vi "Test 2 Degenerate Case Arrangement.vi"(8 "error in (no error)":errorcluster, 11 "Test Case In":refnum<class "Tests.lvclass">) -> (0 "error out":errorcluster, 3 "Test Case Out":refnum<class "Tests.lvclass">)   [LabVIEW 2020, in "Tests.lvclass"]
uses:
  Tests.lvclass
  C:/Program Files (x86)/National Instruments/LabVIEW 2020/vi.lib/Astemes/LUnit/Test Case.lvclass
  <vilib>/Astemes/LUnit/Test Case.lvclass/Test Case.ctl
  4993e8ee-a06a-463a-9684-69129f64d5ce.vi
  <vilib>/Astemes/LUnit/Append Pass Result.vi
  <vilib>/Astemes/LUnit/Append Fail Result.vi
  <vilib>/Astemes/LUnit/Describe Comparison.vi
  <vilib>/Astemes/LUnit/Compare Variants.vi
  <vilib>/Astemes/LUnit/Variant to string.vi
  <vilib>/Utility/Data Type/Get Type Information.vi
  <vilib>/Utility/LVClass/Get LV Class Name.vi
  Proto/Group.lvclass
panel:
  out "Arrangements":u64
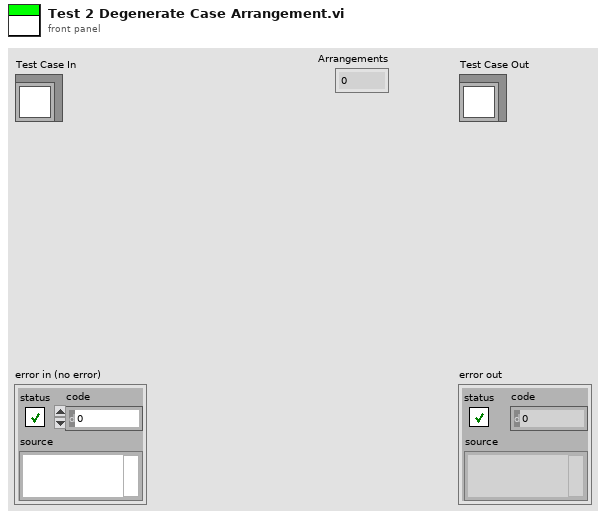
[diagram p1: front panel]
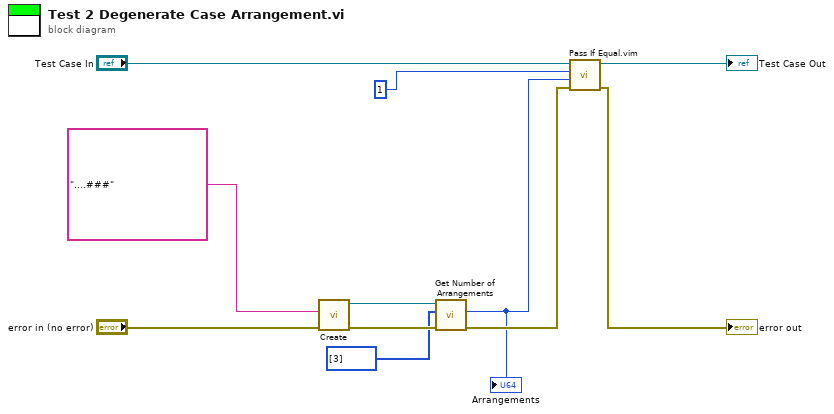
[diagram p0: block diagram]
diagram:
  n1 = call "Create.vi"("error in (no error)"="error in (no error)", "Input"="....###") -> ("error out"=w8:errorcluster, "Group Out"=w6:refnum<class "Group.lvclass">)  [unwired: 8 in]
  n2 = call "Get Number of Arrangements.vi"("error in (no error)"=w8, "Group Sizes"=i64[] [3], "Proto in"=w6) -> ("error out"=w7:errorcluster, "Arrangements"=w4:u64)  [unwired: 6 in, 1 out]
  "Arrangements" <- w4
  n3 = call "Pass If Equal.vim"("error in (no error)"=w7, "Actual"=w4, "Expected"=u64 1 ("Arrangements"), "LUnit Test Case In"="Test Case In") -> ("error out"=→"error out":errorcluster, "LUnit Test Case Out"=→"Test Case Out":refnum<class "Tests.lvclass">)  [unwired: 6 in]
